vi "Lens voltage control.vi"() -> ()   [LabVIEW 2018]
uses:
  <vilib>/Analysis/baseanly.llb/Mean (DBL).vi
  Sub VIs/Save data to file (string).vi
  Sub VIs/Save data to file (double).vi
  <vilib>/Analysis/NI_AALBase.lvlib
panel:
  in  "POWER 2":bool
  out "Voltage divider 2":dbl
  out "Voltage divider 1":dbl
  out "TTL Channels":string[][](array[string])
  out "Ramp Step Size (kV)":dbl=0.025
  out "TDAC voltages":dbl[](array[numeric])
  in  "Active":bool
  in  "Both power supplies at\nsame voltage? (If true, \nPS1 voltage controls both supplies)":bool
  in  "Ramp Voltage?":bool
  in  "PS2 Set Voltage (kV)":dbl min=0.0 max=30.01 step=0.1 format="%.3f"
  in  "PS1 Set Voltage (kV)":dbl min=0.0 max=30.01 step=0.1 format="%.3f"
  in  "Ramp time (s)":dbl=100.0
  out "Polarities":bool[](array[boolean])
  out "Loop iteration time (s)":dbl
  out "Run Time":string="0  00:02:11" caption="Elapsed Time Text"
  out "Supply 2 Current":waveform(dbl)(graph)
  out "Supply 1 Current":waveform(dbl)(graph)
  out "Supply 2 Voltage":waveform(dbl)(graph)
  out "Supply 1 Voltage":waveform(dbl)(graph)
  out "Stream channels":string[][](array[string])
  out "DeviceScanBacklog":i32
  out "LJMScanBacklog":i32=10
  in  "POWER 1":bool
  in  "Polarity switch 2 (ON = pos)":bool
  in  "Polarity switch 1 (ON = pos)":bool
  in  "stop":bool
  in  "Save data path":path
  in  "Save data?":bool caption="Enable"
  out "TDAC channels":string[](array[string])
  out "Actual ScanRate":dbl format="%.2f"
  out "Error Message":string
  in  "Connection Type":string(combo)="ETHERNET_ANY"
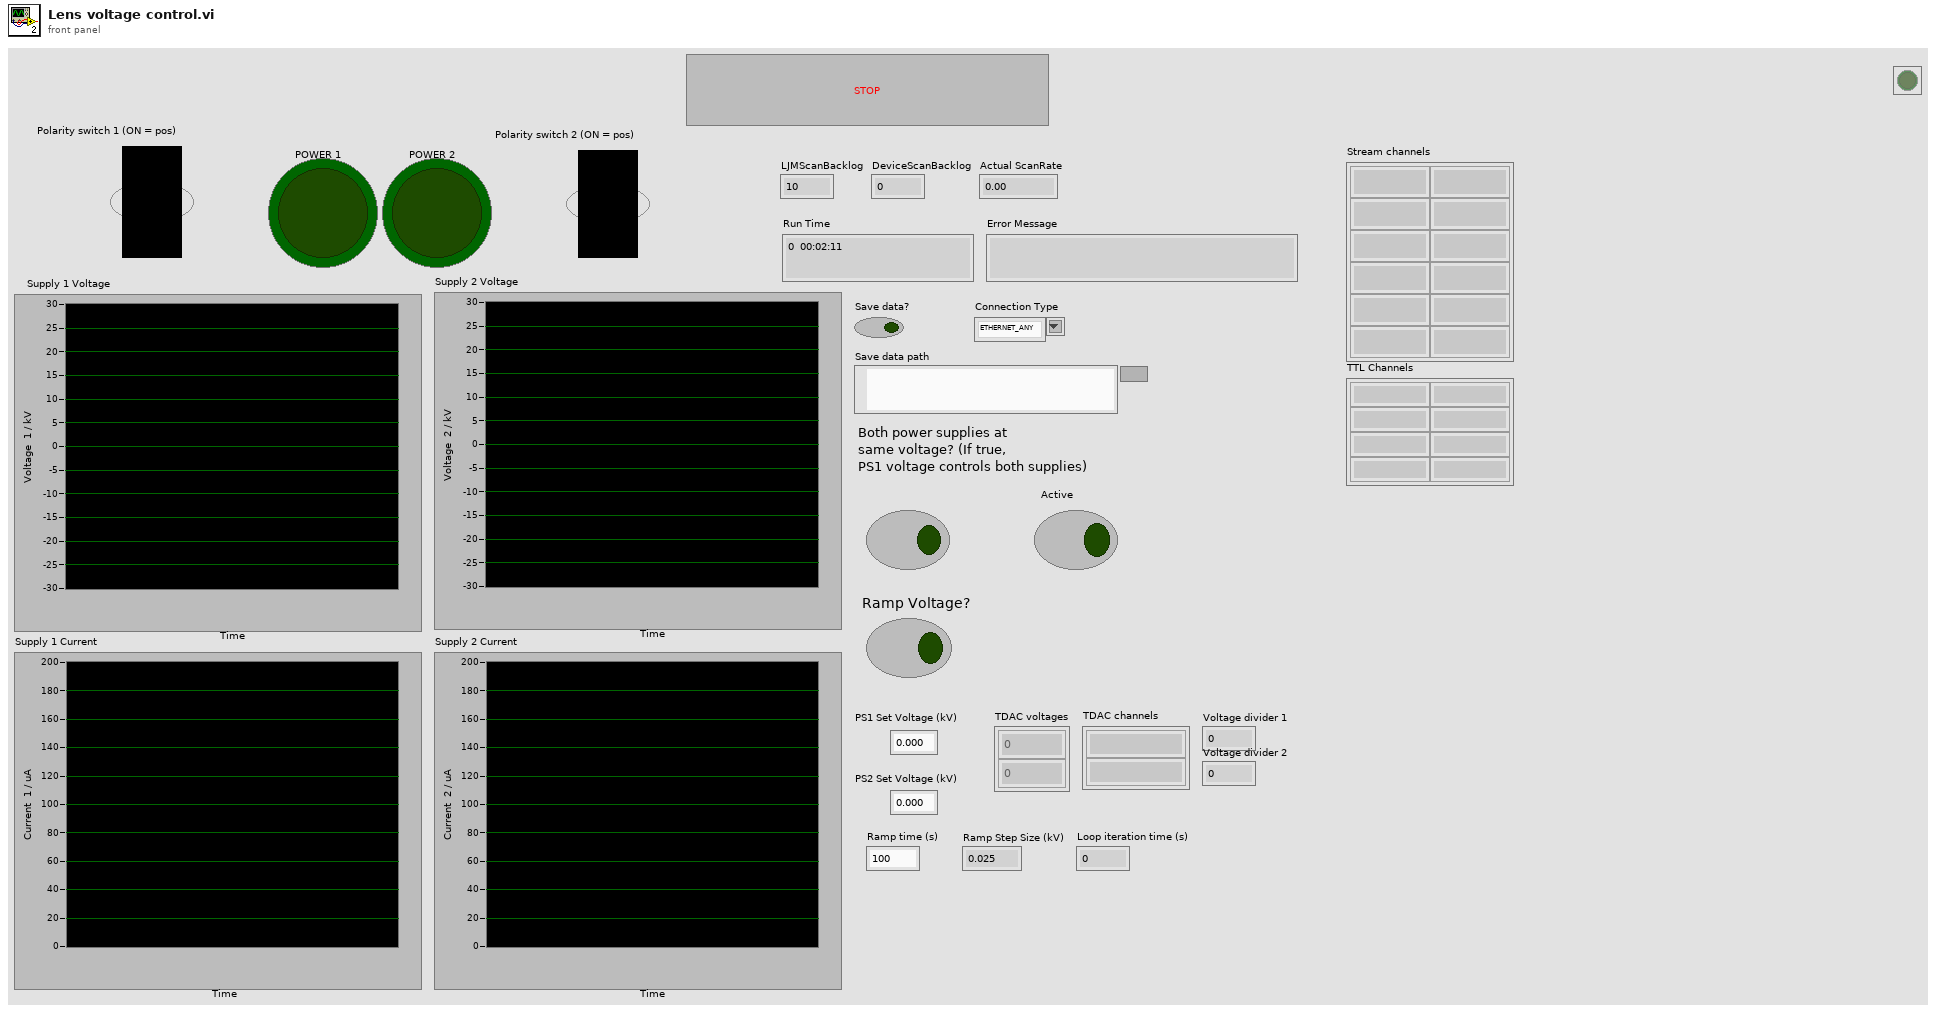
[diagram p1: front panel]
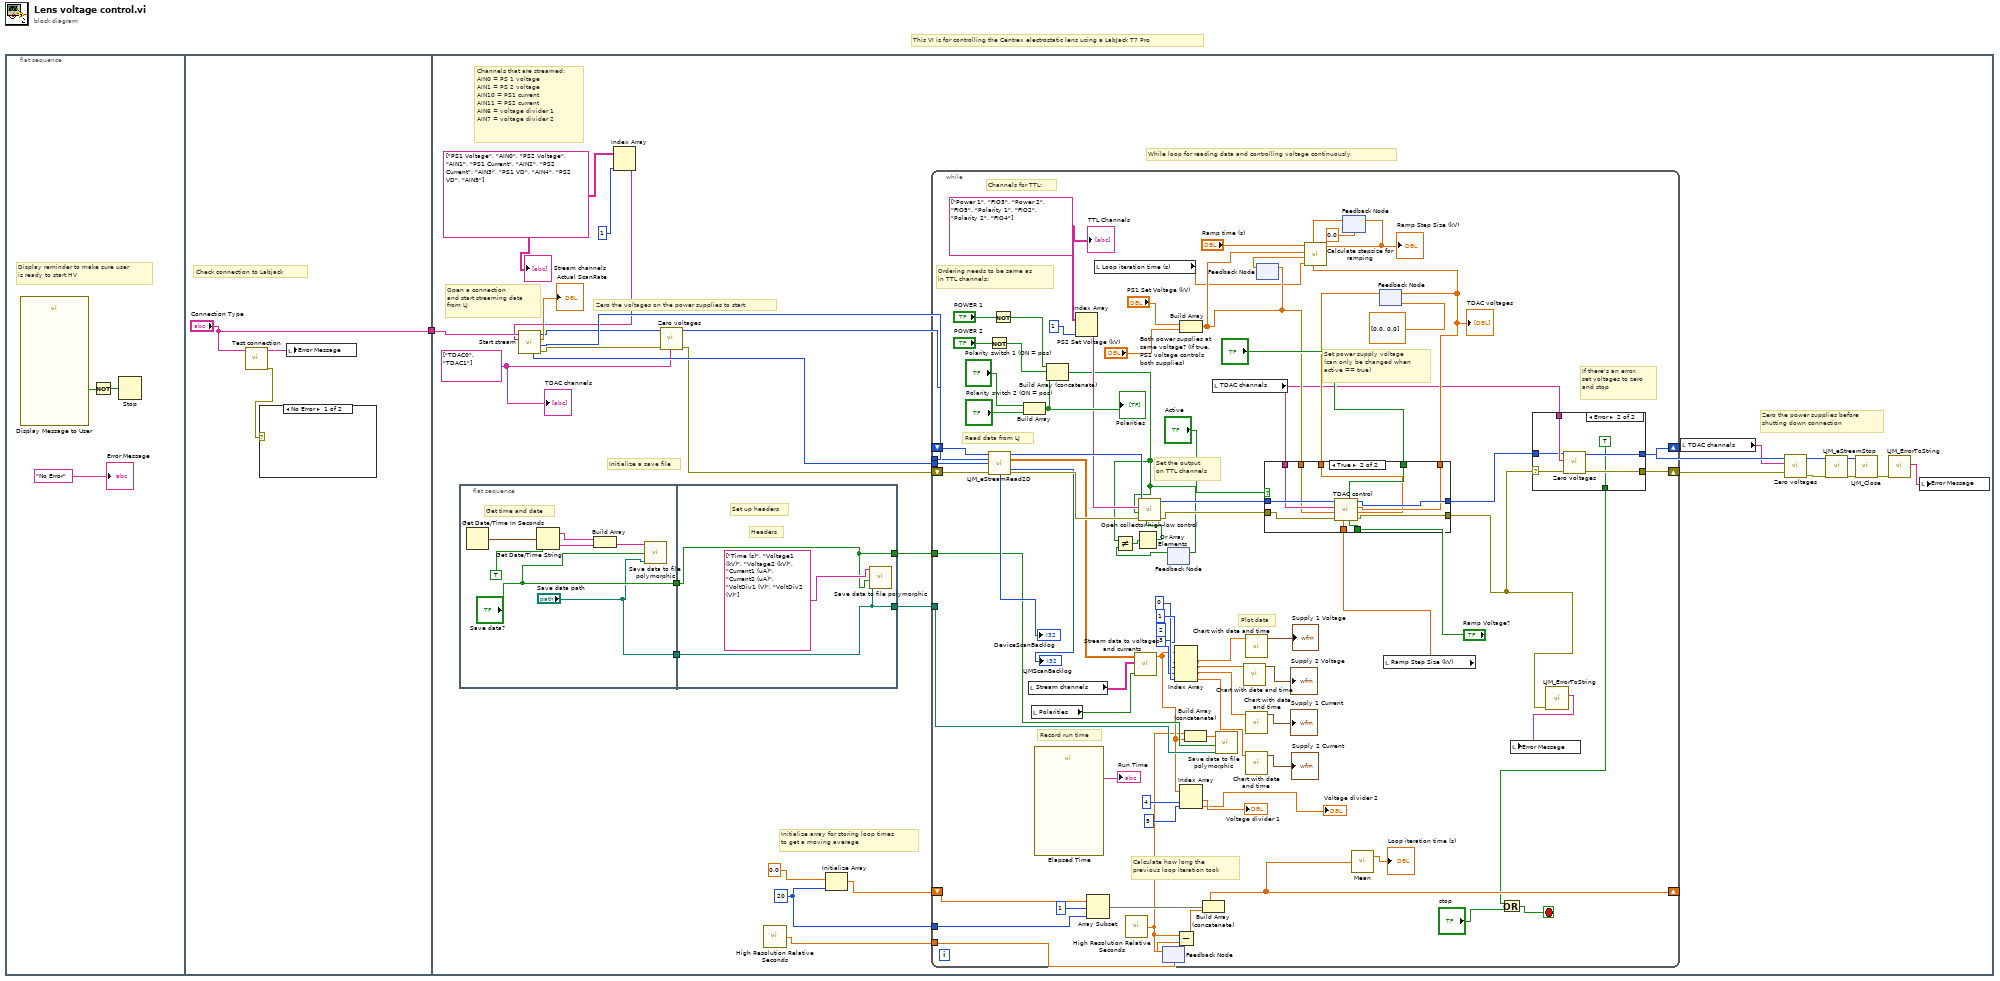
[diagram p0: block diagram]
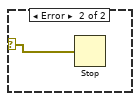
[diagram p2: hidden frame]
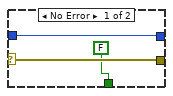
[diagram p3: hidden frame]
diagram:
  # "This VI is for controlling the Centrex electrostatic lens using a LabJack T7 Pro"
  n1 = flat-sequence {
    tunnel: ["Connection Type"] -> w1
    tunnel: w1 -> [w11]
    frame #0 {
      # "Display reminder to make sure user\nis ready to start HV"
      n2 = call "Display Message to User"() -> ("GO GO GO!"=w3:bool)  [unwired: 10 in, 1 out]
      n3 = Not(x=w3) -> (.not. x?=w4:bool)
      n4 = Stop(stop? (T)=w4) -> ()
      "Error Message" <- "No Error" ("Error Message")
    }
    frame #1 {
      # "Check connection to Labjack"
      n5 = call "Test connection.vi"("Connection Type"="Connection Type") -> ("error out"=w5:errorcluster, "Error string"=w7:string)  [unwired: 9 in]
      n6 = case shown="No Error" w5 {
        selector: w5 -> [_ w8]
        frame No Error {
        }
        frame Error {
          n7 = Stop(stop? (T)=w8) -> ()
        }
      }
      n8 = local write "Error Message"(w7) -> ()
    }
    frame #2 {
      w14 = 20
      w13 = string[][] [["PS1 Voltage", "AIN0"], ["PS2 Voltage", "AIN1"], ["PS1 Current", "AIN2"], ["PS2 Current", "AIN3"], ["PS1 VD", "AIN4"], ["PS2 VD", "AIN5"]]
      w12 = string[] ["TDAC0", "TDAC1"]
      # "Initialize array for storing loop times\nto get a moving average"
      # "Zero the power supplies before \nshutting down connection"
      # "Channels that are streamed:\nAIN0 = PS 1 voltage\nAIN1 = PS 2 voltage\nAIN10 = PS1 current\nAIN11 = PS2 current\nAIN6 = voltage divider 1\nAIN7 = voltage divider 2"
      # "While loop for reading data and controlling voltage continuously"
      # "Initialize a save file"
      # "Zero the voltages on the power supplies to start"
      # "Open a connection\nand start streaming data\nfrom LJ"
      n9 = flat-sequence {
        tunnel: ["Save data path"] -> w37
        tunnel: ["Save data?"] -> w36
        tunnel: w37 -> [w152]
        tunnel: w36 -> [w151]
        tunnel: [w152] -> w31
        tunnel: [w151] -> w32
        frame #0 {
          # "Get time and date"
          n10 = Get Date/Time In Seconds() -> (seconds since 1Jan1904=w149:timestamp)
          n11 = Get Date/Time String(seconds (now)=w149, want seconds? (F)=TRUE) -> (date string=w148:string, time string=w147:string)  [unwired: 1 in]
          n12 = Build Array(w148, w147) -> (w146:string[])
          n13 = call-poly "Save data to file polymorphic.vi"("File path"="Save data path", "Save data?"="Save data?", "Data"=w146) -> ()  [unwired: 9 in]
        }
        frame #1 {
          # "Set up headers"
          # "Headers"
          n14 = call-poly "Save data to file polymorphic.vi"("File path"=w152, "Save data?"=w151, "Data"=string[] ["Time (s)", "Voltage1 (kV)", "Voltage2 (kV)", "Current1 (uA)", "Current2 (uA)", "VoltDiv1 (V)", "VoltDiv2 (V)"]) -> ()  [unwired: 9 in]
        }
      }
      n15 = Index Array(array=w13, index (col)=1) -> (element=w10:string[])  [unwired: 1 in]
      n16 = call "Start stream.vi"("Channels to stream"=w10, "Connection type"=w11) -> ("error out"=w17:errorcluster, "ScansPerRead"=w21:i32, "Actual ScanRate"=→"Actual ScanRate":dbl, "Handle out"=w16:i32, "Number of channels"=w22:i32)  [unwired: 5 in]
      n17 = call "Zero voltages.vi"("error in"=w17, "Channels"=w12, "Handle in"=w16) -> ("error out"=w19:errorcluster, "Handle out"=w20:i32)  [unwired: 7 in]
      n18 = call <vilib>:"High Resolution Relative Seconds.vi"() -> ("relative seconds"=w34:dbl)
      n19 = Initialize Array(0.0, w14) -> (w33:dbl[])
      n20 = while {
        tunnel: w21 -> [w118]
        tunnel: w22 -> [w117]
        tunnel: w31 -> [w109]
        tunnel: w32 -> [w108]
        tunnel: w14 -> [w102]
        shift-right: [w97] -> _
        shift-left: w33 -> [w101]
        tunnel: w34 -> [w99]
        shift-right: [w54] -> w23
        shift-left: w19 -> [w120]
        shift-right: [w55] -> w35
        shift-left: w20 -> [w119]
        stop <- w51 stop-if-true
        w64 = string[][] [["Power 1", "FIO3"], ["Power 2", "FIO5"], ["Polarity 1", "FIO2"], ["Polarity 2", "FIO4"]]
        # "Ordering needs to be same as \nin TTL channels:"
        # "If there's an error,\nset voltages to zero\nand stop"
        # "Set power supply voltage\n(can only be changed when\nactive == true)"
        # "Calculate how long the\nprevious loop iteration took"
        # "Record run time"
        # "Plot data"
        # "Set the output \non TTL channels"
        # "Channels for TTL:"
        # "Read data from LJ"
        n21 = Not(x="POWER 2") -> (.not. x?=w40:bool)
        n22 = call "LJM_eStreamRead2D.vi"("Handle In"=w119, "ScansPerRead"=w118, "NumAddresses"=w117, "error in"=w120) -> ("Handle Out"=w116:i32, "aData Out"=w112:dbl[][], "DeviceScanBacklog"=→"DeviceScanBacklog":i32, "LJMScanBacklog"=→"LJMScanBacklog":i32, "error out"=w115:errorcluster)  [unwired: 7 in]
        n23 = Not(x="POWER 1") -> (.not. x?=w39:bool)
        n24 = Build Array("Polarity switch 1 (ON = pos)", "Polarity switch 2 (ON = pos)") -> (w87:bool[])
        "Polarities" <- w87
        n25 = local read "Stream channels"() -> (w111:string[][])
        n26 = local read "Polarities"() -> (w94:bool[])
        n27 = call "Elapsed Time"() -> ("Elapsed Time Text"=→"Run Time":string)  [unwired: 12 in, 7 out]
        n28 = Build Array (concatenate)(w39, w40, w87) -> (w45:bool[])
        n29 = Index Array(array=w64, index (col)=1) -> (element=w66:string[])  [unwired: 1 in]
        n30 = Array Subset(array=w101, index=1, length=w102) -> (w100:dbl[])
        n31 = local read "Loop iteration time (s)"() -> (w82:dbl)
        n32 = call <vilib>:"High Resolution Relative Seconds.vi"() -> ("relative seconds"=w48:dbl)
        n33 = call "Stream data to voltages and currents.vi"("Polarities"=w94, "Stream channels"=w111, "Stream data"=w112) -> ("Data out"=w50:dbl[])  [unwired: 8 in]
        n34 = feedback-in #1(w48) -> ()
        n35 = feedback #1(w99) -> (w95:dbl)
        n36 = feedback-in #2(w45) -> ()
        n37 = feedback #2() -> (w44:bool[])  [unwired: 1 in]
        n38 = Not Equal?(x=w45, y=w44) -> (x != y?=w43:bool[])
        n39 = Or Array Elements(Boolean array=w43) -> (logical OR=w38:bool)
        n40 = call "Open collector high-low control.vi"("Change?"=w38, "error in"=w115, "TTL outputs"=w45, "Channels"=w66, "Handle in"=w116) -> ("error out"=w89:errorcluster, "Handle out"=w90:i32)  [unwired: 5 in]
        n41 = Index Array(array=w50, index #1=0, index #2=1, index #3=2, index #4=3) -> (element #1=w74:dbl, element #2=w73:dbl, element #3=w72:dbl, element #4=w71:dbl)
        n42 = Subtract(x=w48, y=w95) -> (x-y=w98:dbl)
        n43 = Build Array("PS1 Set Voltage (kV)", "PS2 Set Voltage (kV)") -> (w84:dbl[])
        n44 = Index Array(array=w50, index #1=4, index #2=5) -> (element #1=→"Voltage divider 1":dbl, element #2=→"Voltage divider 2":dbl)
        n45 = Build Array (concatenate)(w48, w50) -> (w49:dbl[])
        n46 = Build Array (concatenate)(w100, w98) -> (w97:dbl[])
        n47 = local read "TDAC channels"() -> (w57:string[])
        n48 = call-poly "Save data to file polymorphic.vi"("File path"=w109, "Save data?"=w108, "Data"=w49) -> ()  [unwired: 9 in]
        n49 = call "Chart with date and time.vi"("Data in"=w73) -> ("Waveform Chart"=→"Supply 2 Voltage":waveform(dbl))  [unwired: 10 in]
        n50 = call "Chart with date and time.vi"("Data in"=w74) -> ("Waveform Chart"=→"Supply 1 Voltage":waveform(dbl))  [unwired: 10 in]
        n51 = call "Chart with date and time.vi"("Data in"=w72) -> ("Waveform Chart"=→"Supply 1 Current":waveform(dbl))  [unwired: 10 in]
        n52 = call "Chart with date and time.vi"("Data in"=w71) -> ("Waveform Chart"=→"Supply 2 Current":waveform(dbl))  [unwired: 10 in]
        n53 = feedback-in #3(w84) -> ()
        n54 = feedback #3() -> (w83:dbl[])  [unwired: 1 in]
        n55 = feedback #4(0.0 ("Step size")) -> (w78:dbl)
        n56 = call-poly <vilib>:"Mean.vi"("X"=w97) -> ("mean"=→"Loop iteration time (s)":dbl)  [unwired: 1 out]
        n57 = feedback #5(dbl[] [0.0, 0.0]) -> (w76:dbl[])
        n58 = local read "Ramp Step Size (kV)"() -> (w81:dbl)
        n59 = case shown="True" "Active" {
          tunnel: w90 -> [w132 w143]
          tunnel: w89 -> [w131 w142]
          tunnel: [w131 w141] -> w58
          tunnel: [w132 w140] -> w56
          tunnel: w84 -> [_ w136]
          tunnel: w57 -> [_ w139]
          tunnel: "Both power supplies at\nsame voltage? (If true, \nPS1 voltage controls both supplies)" -> [_ w138]
          tunnel: "Ramp Voltage?" -> [_ w137]
          tunnel: [w130 w135] -> w77
          tunnel: w81 -> [_ w134]
          tunnel: w76 -> [w130 w133]
          frame False {
          }
          frame True {
            n60 = call "TDAC control.vi"("Voltages before"=w133, "Ramp?"=w137, "Same?"=w138, "Step size"=w134, "error in"=w142, "Set voltages"=w136, "Channels"=w139, "Handle in"=w143) -> ("error out"=w141:errorcluster, "TDAC voltages"=w135:dbl[], "Handle out"=w140:i32)  [unwired: 1 in]
          }
        }
        "TDAC voltages" <- w77
        n61 = call "Calculate stepsize for ramping.vi"("TDAC voltages"=w77, "Current step size"=w78, "Loop iteration time"=w82, "Previous set voltages"=w83, "Set voltages"=w84, "Ramp time"="Ramp time (s)") -> ("Step size"=w80:dbl)  [unwired: 5 in]
        "Ramp Step Size (kV)" <- w80
        n62 = feedback-in #4(w80) -> ()
        n63 = feedback-in #5(w77) -> ()
        n64 = case shown="Error" w58 {
          selector: w58 -> [w122 w129]
          tunnel: w57 -> [_ w128]
          tunnel: w56 -> [w123 w127]
          tunnel: [w123 w126] -> w55
          tunnel: [w122 w125] -> w54
          tunnel: [FALSE TRUE] -> w52
          frame No Error {
          }
          frame Error {
            n65 = call "Zero voltages.vi"("error in"=w129, "Channels"=w128, "Handle in"=w127) -> ("error out"=w125:errorcluster, "Handle out"=w126:i32)  [unwired: 7 in]
          }
        }
        n66 = Or(x=w52, y="stop") -> (x .or. y?=w51:bool)
        n67 = call "LJM_ErrorToString.vi"("error in"=w58) -> ("String"=w75:string)  [unwired: 10 in]
        n68 = local write "Error Message"(w75) -> ()
        "TTL Channels" <- w64
      }
      n69 = local read "TDAC channels"() -> (w24:string[])
      n70 = call "Zero voltages.vi"("error in"=w23, "Channels"=w24, "Handle in"=w35) -> ("error out"=w28:errorcluster, "Handle out"=w27:i32)  [unwired: 7 in]
      n71 = call "LJM_eStreamStop.vi"("Handle In"=w27, "error in"=w28) -> ("Handle Out"=w25:i32, "error out"=w26:errorcluster)  [unwired: 12 in]
      n72 = call "LJM_Close.vi"("error in"=w26, "Handle"=w25) -> ("error out"=w30:errorcluster)  [unwired: 9 in]
      n73 = call "LJM_ErrorToString.vi"("error in"=w30) -> ("String"=w29:string)  [unwired: 10 in]
      n74 = local write "Error Message"(w29) -> ()
      "TDAC channels" <- w12
      "Stream channels" <- w13
    }
  }
